vi "初始化前面板对象.vi"(3 "口令":string, 4 "用户名":string) -> (0 "访问权限":string)   [LabVIEW 2010]
panel:
  out "访问确认":bool
  in  "确认":bool
  in  "退出":bool
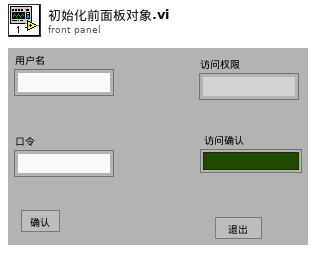
[diagram p1: front panel]
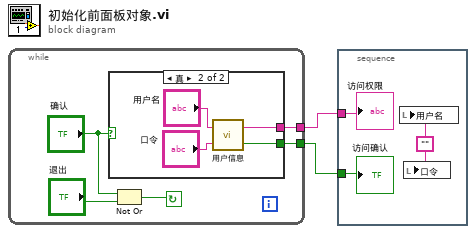
[diagram p0: block diagram]
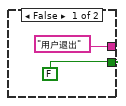
[diagram p2: hidden frame]
diagram:
  n1 = while {
    tunnel: [w4] -> w2
    tunnel: [w3] -> w1
    stop <- w5 continue-if-true
    n2 = case shown="真" "确认" {
      tunnel: ["用户退出" w11] -> w4
      tunnel: [FALSE w10] -> w3
      frame False {
      }
      frame True {
        n3 = call "用户信息.vi"("口令"="口令", "用户名"="用户名") -> ("访问确认"=w10:bool, "访问权限"=w11:string)
      }
    }
    n4 = Not Or(1:"退出", 2:"确认") -> (0:w5:bool)
  }
  n5 = stacked-sequence {
    tunnel: w2 -> [w15]
    tunnel: w1 -> [w14]
    frame #0 {
      w16 = ""
      n6 = local write "用户名"(w16) -> ()
      n7 = local write "口令"(w16) -> ()
      "访问权限" <- w15
      "访问确认" <- w14
    }
  }
